vi "rc_car.vi"() -> ()   [LabVIEW 2019]
panel:
  out "Speed\nIndicator":dbl
  in  "Speed":dbl(slide) scale=-1.0..1.0
  in  "stop":bool
  out "Direction\nIndicator":dbl format="%#_6f"
  in  "Direction":dbl(slide) step=1.0 scale=-1.0..1.0
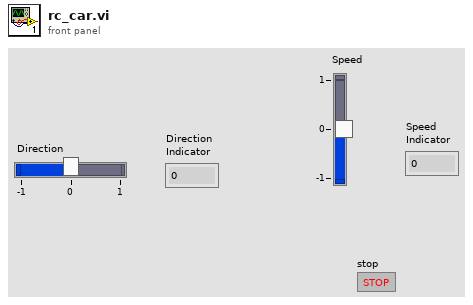
[diagram p1: front panel]
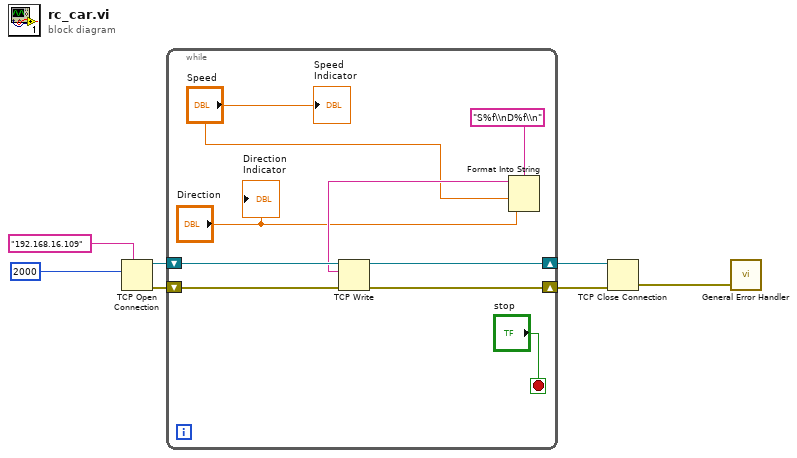
[diagram p0: block diagram]
diagram:
  n1 = TCP Open Connection(address="192.168.16.109", remote port or service name=u16 2000) -> (connection ID=w6:refnum<k5>, error out=w3:errorcluster)  [unwired: 3 in]
  n2 = while {
    shift-right: [w15] -> w5
    shift-left: w6 -> [w16]
    shift-right: [w14] -> w2
    shift-left: w3 -> [w11]
    stop <- "stop" stop-if-true
    n3 = Format Into String(format string="S%f\\nD%f\\n", "Speed", "Direction") -> (resulting string=w10:string)  [unwired: 2 in, 1 out]
    n4 = TCP Write(connection ID=w16, data in=w10, error in (no error)=w11) -> (connection ID out=w15:refnum<k5>, error out=w14:errorcluster)  [unwired: 1 in, 1 out]
    "Direction\nIndicator" <- "Direction"
    "Speed\nIndicator" <- "Speed"
  }
  n5 = TCP Close Connection(connection ID=w5, error in (no error)=w2) -> (error out=w4:errorcluster)  [unwired: 1 in, 1 out]
  n6 = call <vilib>:"General Error Handler.vi"("error in (no error)"=w4) -> ()  [unwired: 10 in, 5 out]
